vi "Lesson5 - array size.vi"() -> ()   [LabVIEW 2013]
panel:
  out "initialized array":string[][][](array[string])
  in  "stop":bool
  in  "disabled index (col)":i32=5
  in  "index (row)":i32=1
  out "concatenated array 2":i32[](array[numeric])
  out "appended array":i32[][](array[numeric])
  out "... pages in layer 5, 4, 3, rows, columns\n(array size incluedes initialized cells only!)":i32[](array[numeric])
  out "element":i32
  in  "Array":dbl[][][][](array[numeric])
  in  "Array - Numeric":dbl[](array[numeric])
  # "click and drag down\non the handle on\nthe row by column\nindicator\nto convert to 2D array"
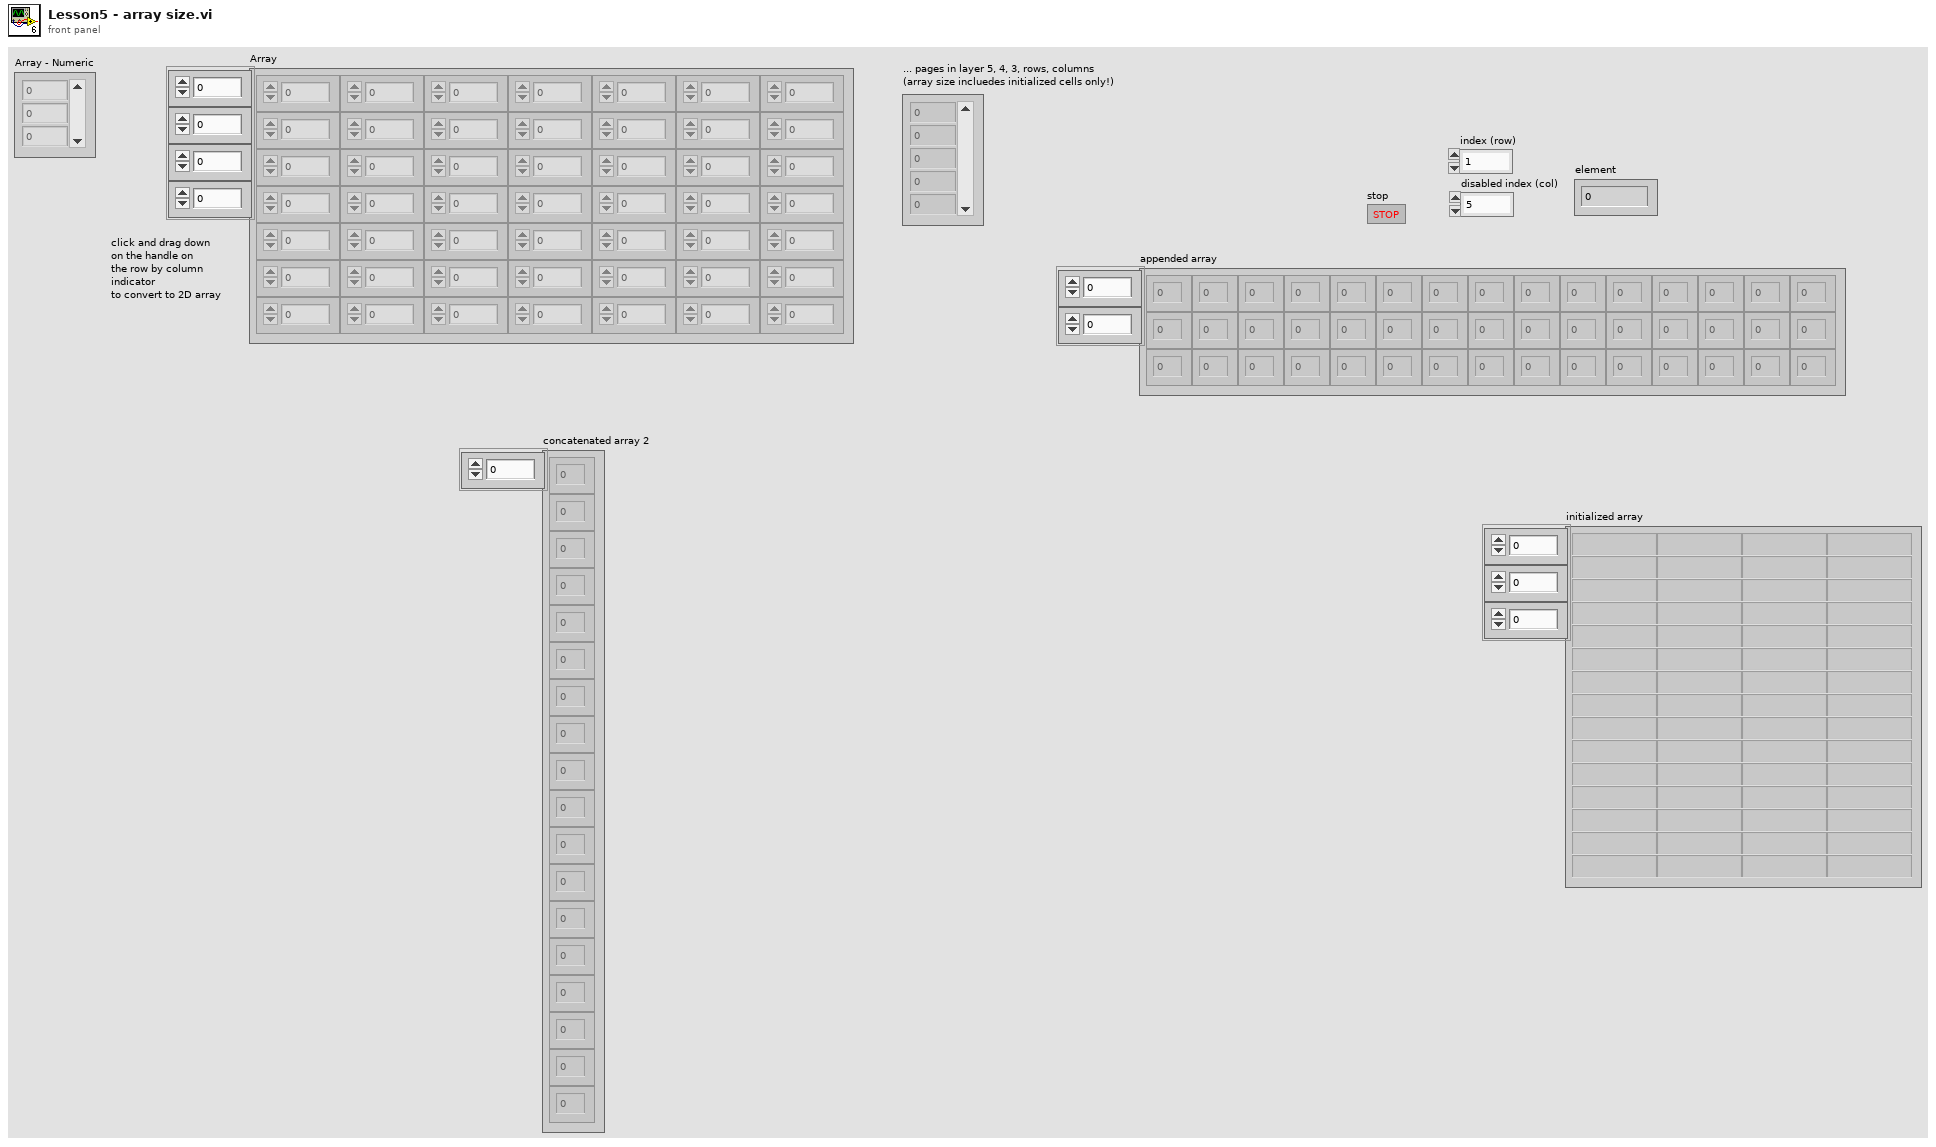
[diagram p1: front panel]
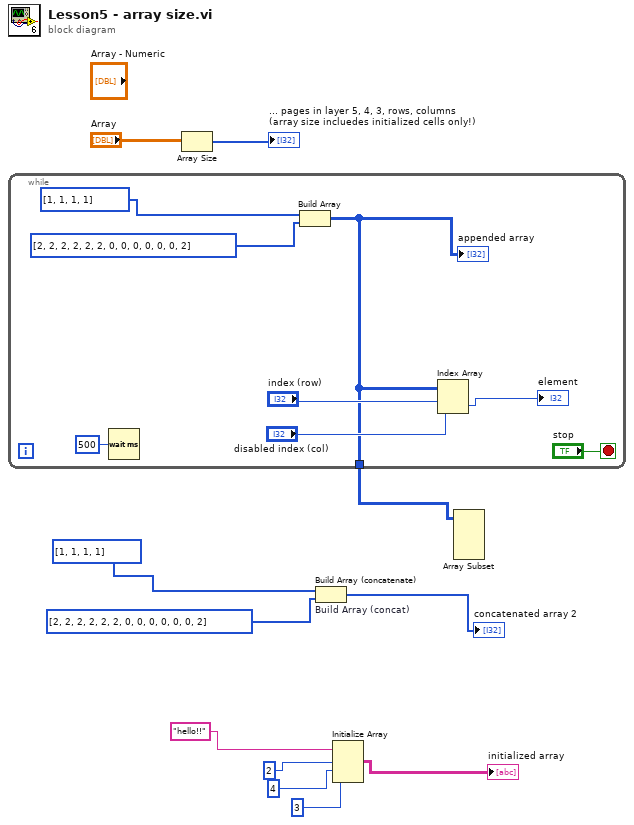
[diagram p0: block diagram]
diagram:
  n1 = while {
    tunnel: [w12] -> w6
    stop <- "stop" stop-if-true
    n2 = Wait (ms)(milliseconds to wait=u32 500) -> ()  [unwired: 1 out]
    n3 = Build Array "Build Array"(i32[] [1, 1, 1, 1], i32[] [2, 2, 2, 2, 2, 2, 0, 0, 0, 0, 0, 0, 2]) -> (w12:i32[][])
    "appended array" <- w12
    n4 = Index Array "Index Array"(array=w12, index (row)="index (row)", index (col)="disabled index (col)") -> (element=→"element":i32)
  }
  n5 = Array Size(array="Array") -> (size(s)=→"... pages in layer 5, 4, 3, rows, columns\n(array size incluedes initialized cells only!)":i32[])
  n6 = Build Array (concatenate) "Build Array (concat)"(i32[] [1, 1, 1, 1], i32[] [2, 2, 2, 2, 2, 2, 0, 0, 0, 0, 0, 0, 2]) -> (→"concatenated array 2":i32[])
  n7 = Initialize Array "Initialize Array"("hello!!", 2, 4, 3) -> (→"initialized array":string[][][])
  n8 = Array Subset "Array Subset"(array=w6) -> ()  [unwired: 4 in, 1 out]
